vi "RT.vi"() -> ()   [LabVIEW 2020]
uses:
  <vilib>/FPGAPlugInAG/cRIO-9054/niLvFpga_Open_cRIO-9054.vi
  <vilib>/Utility/error.llb/Error Cluster From Error Code.vi
  <vilib>/rvi/errors/niLvFpgaAdjustHostInterfaceError.vi
  <vilib>/FPGAPlugInAG/cRIO-9054/niLvFpga_Run_cRIO-9054.vi
  <vilib>/FPGAPlugInAG/cRIO-9054/niLvFpga_Close_cRIO-9054.vi
  <vilib>/rvi/interface/nirviOpenFPGA/nirviOpenFPGA.xnode
  FPGA Bitfiles/basiclogging-fpg_FPGATarget2_FPGA_nEXoHQB2bSM.lvbitx
  FPGA.vi
  <vilib>/rvi/interface/nirviMethod/nirviMethod.xnode
  <vilib>/rvi/interface/nirviReadWriteControl/nirviReadWriteControl.xnode
  <vilib>/rvi/interface/nirviCloseFPGA/nirviCloseFPGA.xnode
  <vilib>/rvi/errors/niLvFpgaMergeErrorWithErrorCode.vi
  <vilib>/FPGAPlugInAG/cRIO-9054/niLvFpga_StartFifo_cRIO-9054.vi
  NiFpgaLv.dll
  <vilib>/FPGAPlugInAG/cRIO-9054/niLvFpga_ReadFifo_cRIO-9054.vi
panel:
  out "Waveform Chart":dbl[][](graph)
  out "size(s)":i32[](array[numeric])
  out "output array":dbl[][](array[numeric])
  out "Data":fxp<+/-,24,7>[](array[numeric]) format="%.20g"
  out "error out":errorcluster
  out "Timed Out?":bool
  out "Analog Input Chart":dbl[][](graph)
  in  "Loop rate (uSec)":u32=500
  in  "stop":bool
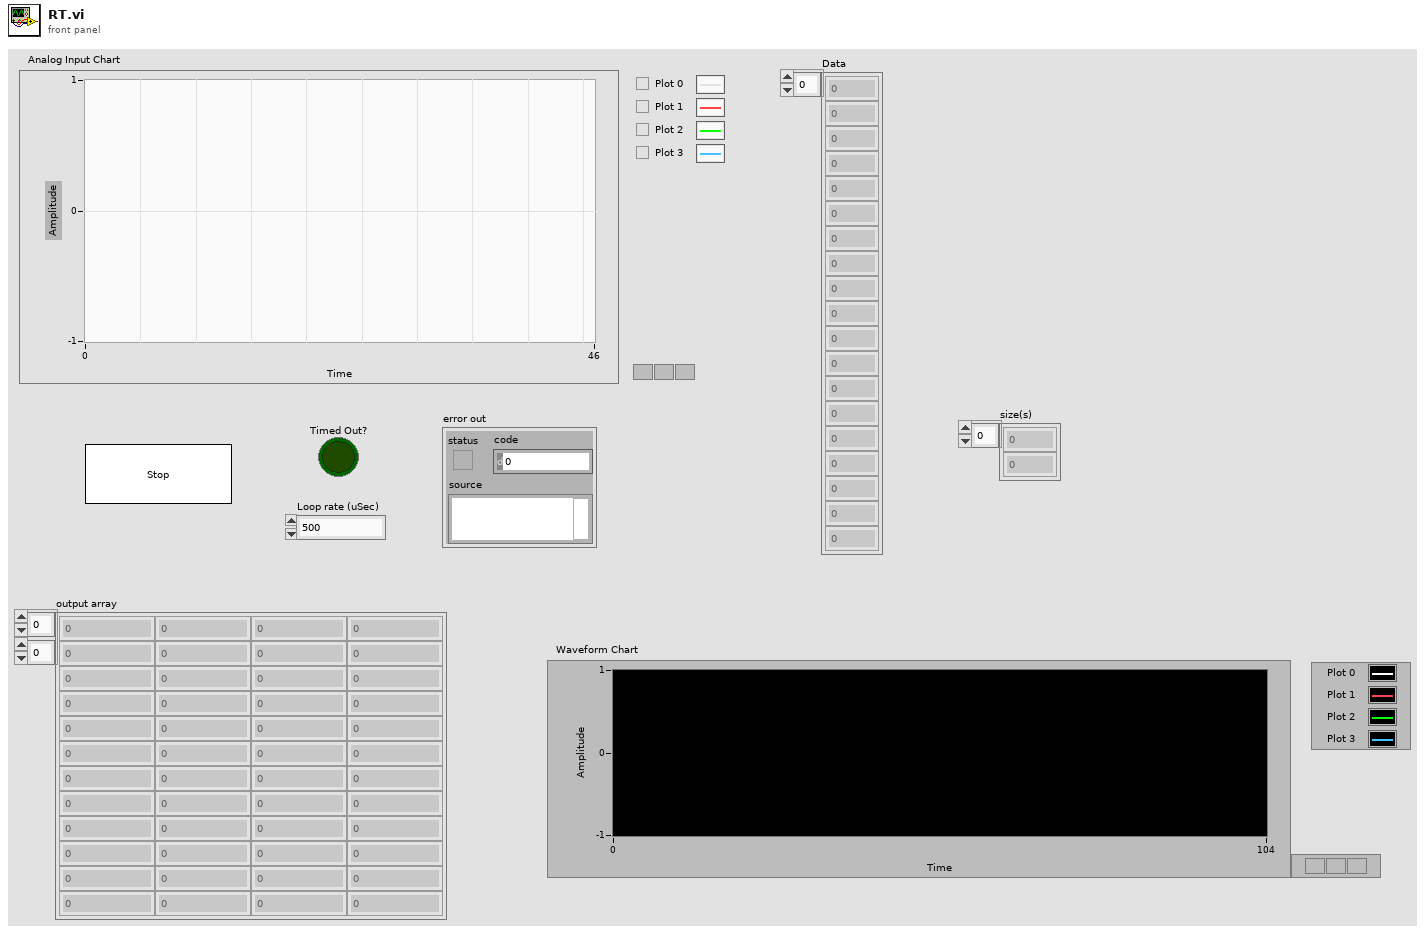
[diagram p1: front panel]
types:
  T1 = enum16{"open", "open or create", "create or replace", "create", "open (read-only)"}
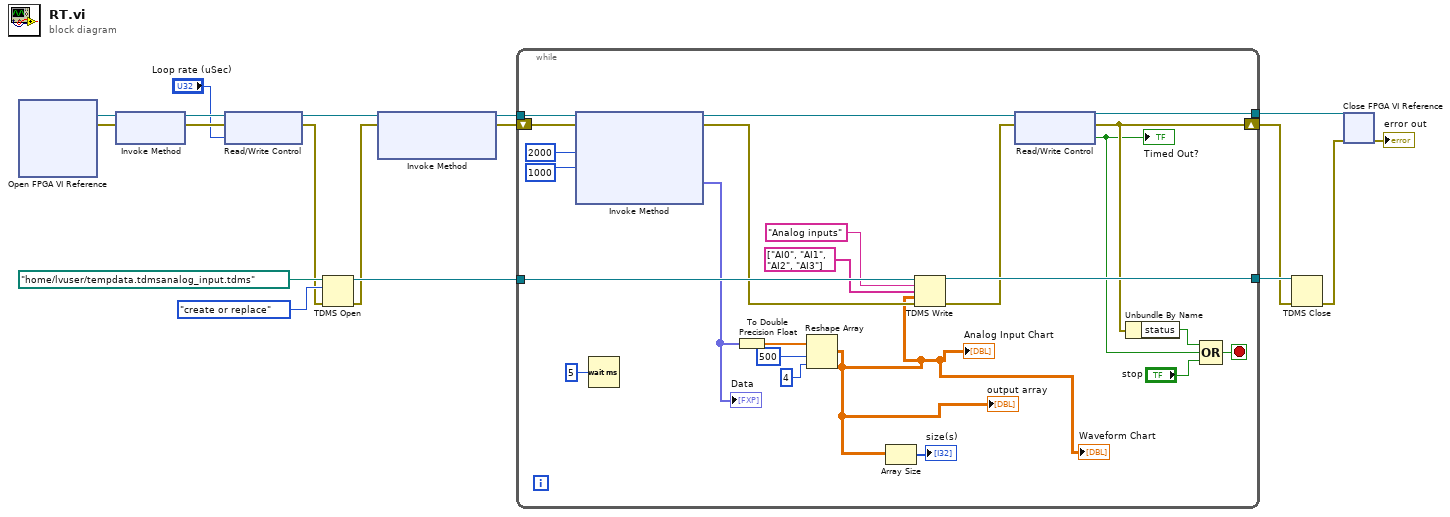
[diagram p0: block diagram]
diagram:
  n1 = xnode "Open FPGA VI Reference"() -> ("FPGA VI Reference Out"=w8:refnum<k20>, "error out"=w7:errorcluster)  [unwired: 2 in]
  n2 = xnode "Invoke Method"("FPGA VI Reference In"=w8, "error in"=w7) -> ("FPGA VI Reference Out"=w15:refnum<k20>, "error out"=w13:errorcluster)
  n3 = xnode "Read/Write Control"("FPGA VI Reference In"=w15, "error in"=w13, "Rate (uSec)"="Loop rate (uSec)") -> ("FPGA VI Reference Out"=w14:refnum<k20>, "error out"=w5:errorcluster)
  n4 = TDMS Open(8:w5, 10:T1."create or replace" ("operation (0:open)"), 11:path "/home/lvuser/tempdata.tdmsanalog_input.tdms" ("file path")) -> (0:w4:errorcluster, 3:w16:refnum<k34>)  [unwired: 4 in]
  n5 = xnode "Invoke Method"("FPGA VI Reference In"=w14, "error in"=w4) -> ("FPGA VI Reference Out"=w18:refnum<k20>, "error out"=w9:errorcluster)  [unwired: 1 in]
  n6 = while {
    tunnel: w18 -> [w42]
    tunnel: [w32] -> w6
    tunnel: [w36] -> w17
    tunnel: w16 -> [w35]
    shift-right: [w24] -> w3
    shift-left: w9 -> [w41]
    stop <- w31 stop-if-true
    n7 = xnode "Invoke Method"("FPGA VI Reference In"=w42, "error in"=w41, "Number of Elements"=u32 2000, "Timeout (ms)"=1000) -> ("FPGA VI Reference Out"=w28:refnum<k20>, "error out"=w23:errorcluster, "Data"=w27:fxp<+/-,24,7>[])  [unwired: 1 out]
    "Data" <- w27
    n8 = Wait (ms)(milliseconds to wait=u32 5) -> ()  [unwired: 1 out]
    n9 = To Double Precision Float(number=w27) -> (double precision float=w29:dbl[])
    n10 = Reshape Array(w29, 500 ("dimension size"), 4 ("dimension size")) -> (w19:dbl[][])
    "Analog Input Chart" <- w19
    "output array" <- w19
    "Waveform Chart" <- w19
    n11 = Array Size(array=w19) -> (size(s)=→"size(s)":i32[])
    n12 = TDMS Write(0:w35, 5:"Analog inputs" ("group name in (Untitled)"), 7:string[] ["AI0", "AI1", "AI2", "AI3"] ("channel name(s) in (Untitled)"), 9:w19, 11:w23) -> (4:w36:refnum<k34>, 15:w22:errorcluster)  [unwired: 1 in, 2 out]
    n13 = xnode "Read/Write Control"("FPGA VI Reference In"=w28, "error in"=w22) -> ("FPGA VI Reference Out"=w32:refnum<k20>, "error out"=w24:errorcluster, "Timed Out?"=w21:bool)
    "Timed Out?" <- w21
    n14 = Unbundle By Name(w24) -> ("status"=w26:bool)
    n15 = Compound Arithmetic op=OR(w26, w21, "stop") -> (w31:bool)
  }
  n16 = TDMS Close(8:w3, 11:w17) -> (0:w2:errorcluster)  [unwired: 1 out]
  n17 = xnode "Close FPGA VI Reference"("FPGA VI Reference In"=w6, "error in"=w2) -> ("error out"=→"error out":errorcluster)
